vi "CCE T027 SubVI06.vi"(11 "Image Data":u8[][](array[numeric])) -> (3 "HU":dbl[](array[numeric]))   [LabVIEW 2020]
doc: "Ceballos Conde Emanuel 4MV6 Sistemas de visión artificial 2022/1\neste vi permite obtener los 7 momentos de Hu ingrsando una imagen previamente binarizada"
panel:
  out "hu7":dbl
  out "hu6":dbl
  out "hu5":dbl
  out "hu4":dbl
  out "hu3":dbl
  out "hu2":dbl
  out "hu1":dbl
  # "Ceballos Conde Emanuel\n4MV6\nSistemas de visión artificial\n2022/1"
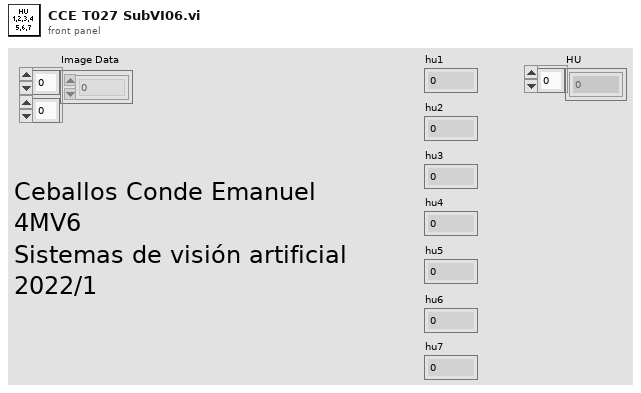
[diagram p1: front panel]
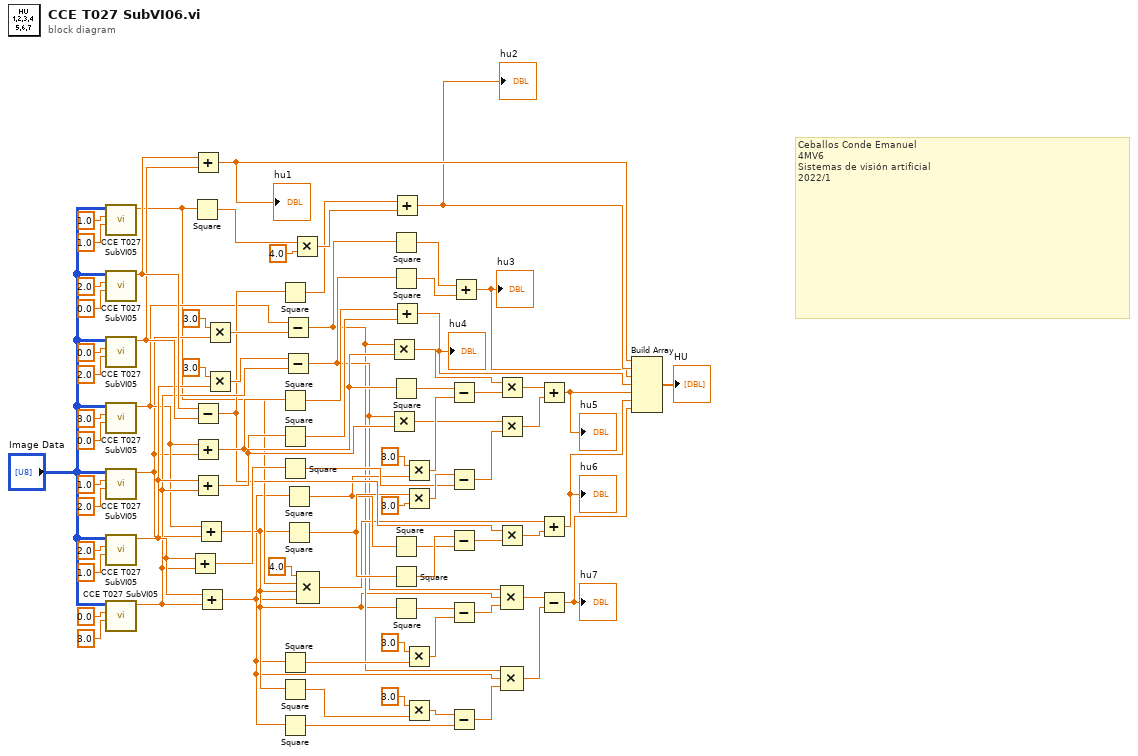
[diagram p0: block diagram]
diagram:
  # "Ceballos Conde Emanuel\n4MV6\nSistemas de visión artificial\n2022/1"
  n1 = call "CCE T027 SubVI05.vi"("q"=1.0, "p"=1.0, "Image Data"="Image Data") -> ("m normalizado"=w26:dbl)  [unwired: 8 in]
  n2 = call "CCE T027 SubVI05.vi"("q"=0.0, "p"=2.0, "Image Data"="Image Data") -> ("m normalizado"=w62:dbl)  [unwired: 8 in]
  n3 = call "CCE T027 SubVI05.vi"("q"=2.0, "p"=0.0, "Image Data"="Image Data") -> ("m normalizado"=w61:dbl)  [unwired: 8 in]
  n4 = call "CCE T027 SubVI05.vi"("q"=0.0, "p"=3.0, "Image Data"="Image Data") -> ("m normalizado"=w33:dbl)  [unwired: 8 in]
  n5 = call "CCE T027 SubVI05.vi"("q"=2.0, "p"=1.0, "Image Data"="Image Data") -> ("m normalizado"=w32:dbl)  [unwired: 8 in]
  n6 = call "CCE T027 SubVI05.vi"("q"=1.0, "p"=2.0, "Image Data"="Image Data") -> ("m normalizado"=w43:dbl)  [unwired: 8 in]
  n7 = call "CCE T027 SubVI05.vi"("q"=3.0, "p"=0.0, "Image Data"="Image Data") -> ("m normalizado"=w42:dbl)  [unwired: 8 in]
  n8 = Add(x=w43, y=w42) -> (x+y=w41:dbl)
  n9 = Square(x=w26) -> (x^2=w9:dbl)
  n10 = Add(x=w62, y=w61) -> (x+y=w8:dbl)
  "hu1" <- w8
  n11 = Subtract(x=w62, y=w61) -> (x-y=w37:dbl)
  n12 = Add(x=w33, y=w32) -> (x+y=w54:dbl)
  n13 = Add(x=w43, y=w42) -> (x+y=w47:dbl)
  n14 = Add(x=w33, y=w32) -> (x+y=w11:dbl)
  n15 = Add(x=w43, y=w42) -> (x+y=w10:dbl)
  n16 = Multiply(x=3.0, y=w32) -> (x*y=w63:dbl)
  n17 = Multiply(x=3.0, y=w43) -> (x*y=w59:dbl)
  n18 = Square(x=w37) -> (x^2=w74:dbl)
  n19 = Square(x=w54) -> (x^2=w56:dbl)
  n20 = Square(x=w47) -> (x^2=w55:dbl)
  n21 = Square(x=w41) -> (x^2=w40:dbl)
  n22 = Square(x=w10) -> (x^2=w20:dbl)
  n23 = Square(x=w11) -> (x^2=w13:dbl)
  n24 = Square(x=w10) -> (x^2=w12:dbl)
  n25 = Subtract(x=w33, y=w63) -> (x-y=w17:dbl)
  n26 = Subtract(x=w59, y=w42) -> (x-y=w25:dbl)
  n27 = Square(x=w10) -> (x^2=w30:dbl)
  n28 = Square(x=w11) -> (x^2=w31:dbl)
  n29 = Multiply(x=w9, y=4.0) -> (x*y=w75:dbl)
  n30 = Compound Arithmetic op=MULTIPLY(4.0 ("value"), w26, w11, w10) -> (w28:dbl)
  n31 = Multiply(x=w17, y=w54) -> (x*y=w50:dbl)
  n32 = Multiply(x=w25, y=w47) -> (x*y=w46:dbl)
  n33 = Square(x=w17) -> (x^2=w58:dbl)
  n34 = Square(x=w25) -> (x^2=w57:dbl)
  n35 = Square(x=w54) -> (x^2=w53:dbl)
  n36 = Square(x=w30) -> (x^2=w34:dbl)
  n37 = Square(x=w31) -> (x^2=w35:dbl)
  n38 = Square(x=w11) -> (x^2=w23:dbl)
  n39 = Add(x=w74, y=w75) -> (x+y=w7:dbl)
  "hu2" <- w7
  n40 = Add(x=w56, y=w55) -> (x+y=w5:dbl)
  "hu4" <- w5
  n41 = Multiply(x=3.0, y=w30) -> (x*y=w52:dbl)
  n42 = Multiply(x=w31, y=3.0) -> (x*y=w44:dbl)
  n43 = Multiply(x=3.0, y=w20) -> (x*y=w22:dbl)
  n44 = Multiply(x=3.0, y=w13) -> (x*y=w14:dbl)
  n45 = Subtract(x=w53, y=w52) -> (x-y=w49:dbl)
  n46 = Subtract(x=w44, y=w40) -> (x-y=w39:dbl)
  n47 = Subtract(x=w35, y=w34) -> (x-y=w36:dbl)
  n48 = Subtract(x=w23, y=w22) -> (x-y=w24:dbl)
  n49 = Subtract(x=w14, y=w12) -> (x-y=w16:dbl)
  n50 = Add(x=w58, y=w57) -> (x+y=w6:dbl)
  "hu3" <- w6
  n51 = Multiply(x=w50, y=w49) -> (x*y=w48:dbl)
  n52 = Multiply(x=w46, y=w39) -> (x*y=w38:dbl)
  n53 = Multiply(x=w37, y=w36) -> (x*y=w29:dbl)
  n54 = Compound Arithmetic op=MULTIPLY(w25, w11, w24) -> (w19:dbl)
  n55 = Compound Arithmetic op=MULTIPLY(w17, w10, w16) -> (w18:dbl)
  n56 = Add(x=w48, y=w38) -> (x+y=w4:dbl)
  "hu5" <- w4
  n57 = Add(x=w28, y=w29) -> (x+y=w3:dbl)
  "hu6" <- w3
  n58 = Subtract(x=w19, y=w18) -> (x-y=w2:dbl)
  "hu7" <- w2
  n59 = Build Array(w8, w7, w6, w5, w4, w3, w2) -> (→"HU":dbl[])
